vi "PXI-Find Counter Devices.vi"(7 "Direction":enum16{"Output", "Input", "Either"}(ring), 11 "error in (no error)":errorcluster) -> (4 "CTR channels":tag[](array[tag]), 15 "error out":errorcluster)   [LabVIEW 2020]
uses:
  <resource>/objmgr/daqmx.rc
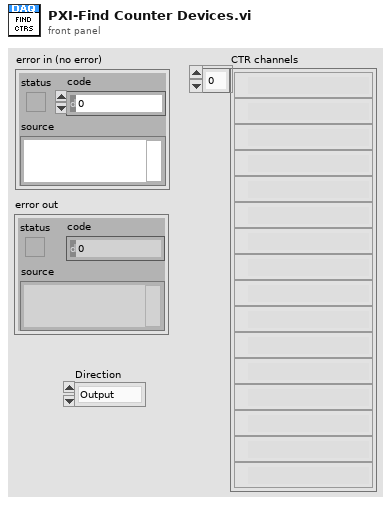
[diagram p1: front panel]
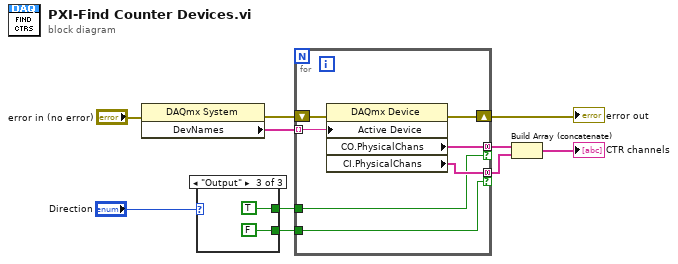
[diagram p0: block diagram]
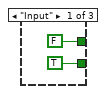
[diagram p2: hidden frame]
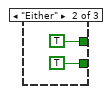
[diagram p3: hidden frame]
diagram:
  n1 = property class="DAQmx System"(error in="error in (no error)") -> (error out=w8:errorcluster, "DevNames"=w9:tag[])  [unwired: 1 in, 1 out]
  n2 = case shown="\"Output\"" "Direction" {
    tunnel: [FALSE TRUE TRUE] -> w5
    tunnel: [TRUE TRUE FALSE] -> w1
    frame "Input" {
    }
    frame "Either" {
    }
    frame "Output" {
    }
  }
  n3 = for {
    tunnel: w9 -> [w22] mode=indexing
    shift-right: [w23] -> w7
    shift-left: w8 -> [w21]
    tunnel: [w20] -> w4 mode=concatenating if=w18
    tunnel: [w19] -> w3 mode=concatenating if=w17
    tunnel: w5 -> [w18]
    tunnel: w1 -> [w17]
    n4 = property class="DAQmx Device"(error in=w21, "Active Device"=w22) -> (error out=w23:errorcluster, "CO.PhysicalChans"=w20:tag[], "CI.PhysicalChans"=w19:tag[])  [unwired: 1 in, 1 out]
  }
  "error out" <- w7
  n5 = Build Array (concatenate)(w4, w3) -> (→"CTR channels":tag[])
